vi "read.vi"(8 "error in (no error)":errorcluster caption="错误输入（无错误）", 11 "serial 输入":refnum<class "serial.lvclass">) -> (0 "error out":errorcluster caption="错误输出", 2 "read":string, 3 "serial 输出":refnum<class "serial.lvclass">)   [LabVIEW 2016, in "潮位站数据传输.lvlib" / "serial.lvclass"]
uses:
  serial.lvclass
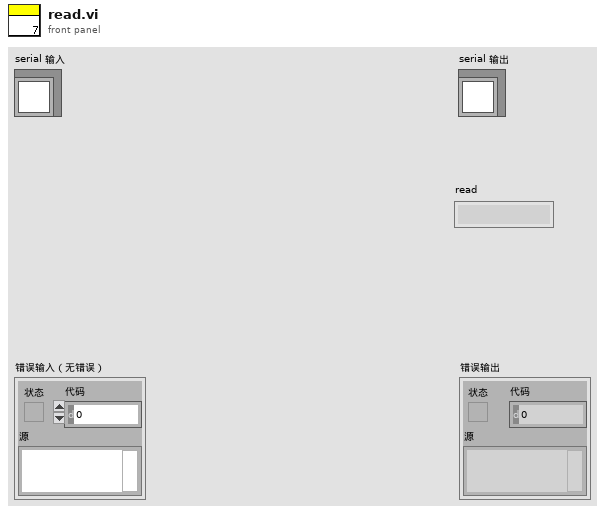
[diagram p1: front panel]
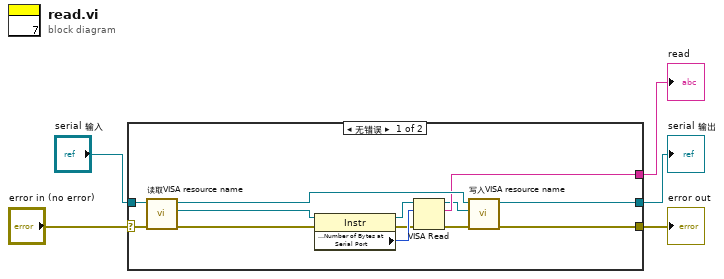
[diagram p0: block diagram]
diagram:
  n1 = case shown="无错误" "error in (no error)" {
    selector: "error in (no error)" -> [w14 w19]
    tunnel: "serial 输入" -> [w15 w20]
    tunnel: [w10 _] -> w3
    tunnel: [w7 w19] -> w2
    tunnel: [w6 w20] -> w1
    frame No Error {
      n2 = call-dynamic "读取VISA resource name.vi"("error in (no error)"=w14, "data_inter输入"=w15) -> ("error out"=w13:errorcluster, "VISA resource name"=w12:refnum<visa-resource-name>, "data_inter输出"=w11:refnum<class "serial.lvclass">)  [unwired: 7 in]
      n3 = property class="Instr"(reference=w12, error in=w13) -> (reference out=w16:refnum<visa-resource-name>, error out=w17:errorcluster, "Serial Settings:Number of Bytes at Serial Port"=w18:u32)
      n4 = VISA Read(VISA resource name=w16, byte count=w18, error in (no error)=w17) -> (VISA resource name out=w9:refnum<visa-resource-name>, read buffer=w10:string, error out=w8:errorcluster)  [unwired: 1 out]
      n5 = call-dynamic "写入VISA resource name.vi"("error in (no error)"=w8, "VISA resource name"=w9, "data_inter输入"=w11) -> ("error out"=w7:errorcluster, "data_inter输出"=w6:refnum<class "serial.lvclass">)  [unwired: 7 in]
    }
    frame Error {
    }
  }
  "error out" <- w2
  "serial 输出" <- w1
  "read" <- w3
